vi "Send Immediate Trigger.vi"(7 "Device Action (2: Both)":i32(ring)=2 items=["Acquire", "Transient", "Both"], 8 "error in (no error)":errorcluster, 9 "Trigger Type (0: Arm Trigger)":i32(ring) items=["Arm Trigger", "Normal Trigger"], 10 "Channel (1: Channel 1)":i32(ring)=1 items=["Channel 1"=1], 11 "VISA resource name":refnum<visa-resource-name>) -> (0 "error out":errorcluster, 3 "VISA resource name out":refnum<visa-resource-name>)   [LabVIEW 2012, in "Keysight B2980 Series.lvlib"]
doc: "Sends an immediate arm trigger or a normal trigger for the specified device action to the specified channel."
uses:
  Keysight B2980 Series.lvlib
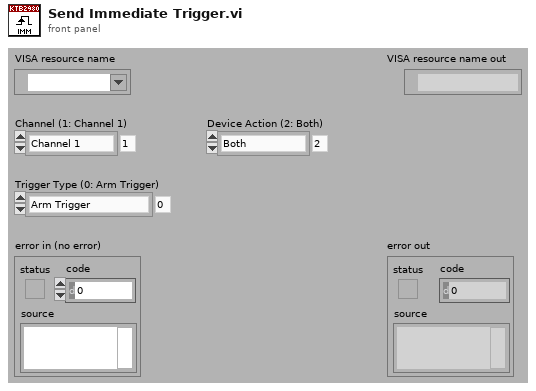
[diagram p1: front panel]
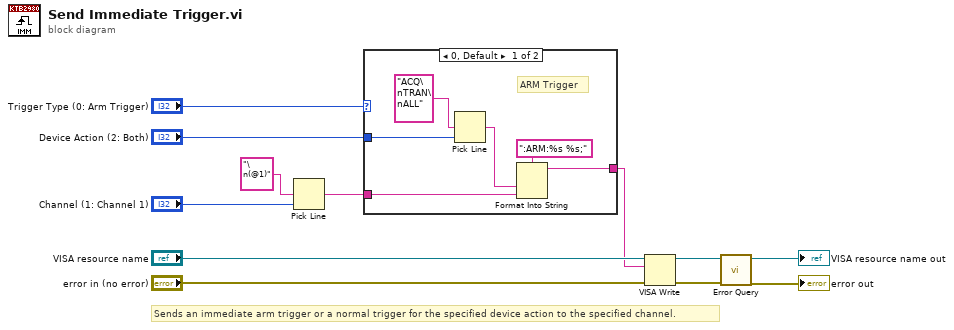
[diagram p0: block diagram]
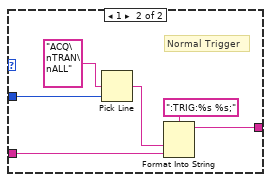
[diagram p2: hidden frame]
diagram:
  # "Sends an immediate arm trigger or a normal trigger for the specified device action to the specified channel."
  n1 = Pick Line(multi-line string="\n(@1)", line index="Channel (1: Channel 1)") -> (output string=w3:string)  [unwired: 1 out]
  n2 = case shown="0, Default" "Trigger Type (0: Arm Trigger)" {
    tunnel: w3 -> [w15 w20]
    tunnel: "Device Action (2: Both)" -> [w14 w19]
    tunnel: [w13 w21] -> w1
    frame 0, Default {
      # "ARM Trigger"
      n3 = Pick Line(multi-line string="ACQ\nTRAN\nALL", line index=w14) -> (output string=w16:string)  [unwired: 1 out]
      n4 = Format Into String(format string=":ARM:%s %s;", w16, w15) -> (resulting string=w13:string)  [unwired: 2 in, 1 out]
    }
    frame 1 {
      # "Normal Trigger"
      n5 = Pick Line(multi-line string="ACQ\nTRAN\nALL", line index=w19) -> (output string=w22:string)  [unwired: 1 out]
      n6 = Format Into String(format string=":TRIG:%s %s;", w22, w20) -> (resulting string=w21:string)  [unwired: 2 in, 1 out]
    }
  }
  n7 = VISA Write(VISA resource name="VISA resource name", write buffer=w1, error in (no error)="error in (no error)") -> (VISA resource name out=w10:refnum<visa-resource-name>, error out=w9:errorcluster)  [unwired: 1 out]
  n8 = call "Error Query.vi"("error in (no error)"=w9, "VISA resource name"=w10) -> ("error out"=→"error out":errorcluster, "VISA resource name out"=→"VISA resource name out":refnum<visa-resource-name>)  [unwired: 8 out]
